vi "Subsequence Exchange Crossover(SXX).vi"(8 "Number of Jobs":i32, 9 "Number of Machines":i32, 10 "Schedule 2":u16[](array[numeric]), 11 "Schedule 1":u16[](array[numeric])) -> (2 "Child 2":T1, 3 "Child 1":T1)   [LabVIEW 2013, in "GA.lvclass"]
uses:
  GA.lvclass
  Controls/Subsequence.ctl
  Controls/Appropraite Subsequences for SXX.ctl
  Controls/Solution_GA.ctl
  <vilib>/Analysis/NI_AALBase.lvlib
  <vilib>/Analysis/1siggen.llb/Riffle Array (I32).vi
panel:
  out "Schedule 2":u16[](array[numeric])
  out "Schedule 1":u16[](array[numeric])
  out "Appropriate Subsequences":T2[](array[typedef])
  out "All Subarrays Out 2":T3[](array[typedef])
  out "All Subarrays Out 1":T3[](array[typedef])
  out "JO4M Sch2":u16[][](array[numeric])
  out "JO4M Sch1":u16[][](array[numeric])
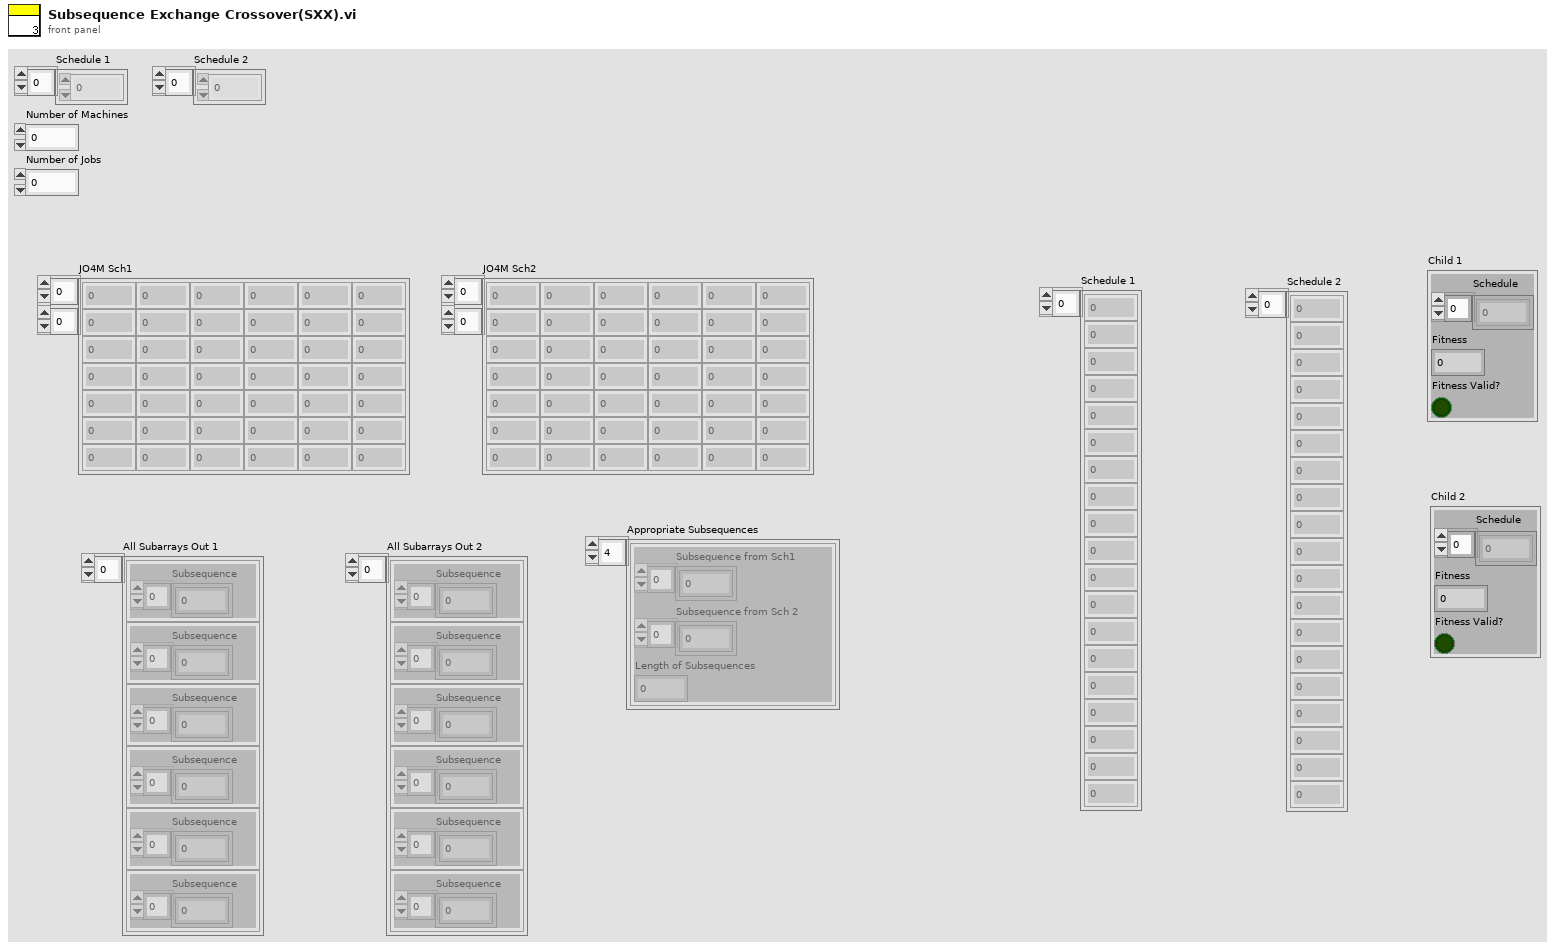
[diagram p1: front panel]
types:
  T1 = typedef "Solution_GA.ctl" = cluster{"Schedule":u16[], "Fitness":u16, "Fitness Valid?":bool}
  T2 = typedef "Appropraite Subsequences for SXX.ctl" = cluster{"Subsequence from Sch1":i32[], "Subsequence from Sch 2":i32[], "Length of Subsequences":i32}
  T3 = typedef "Subsequence.ctl" = cluster{"Subsequence":i32[]}
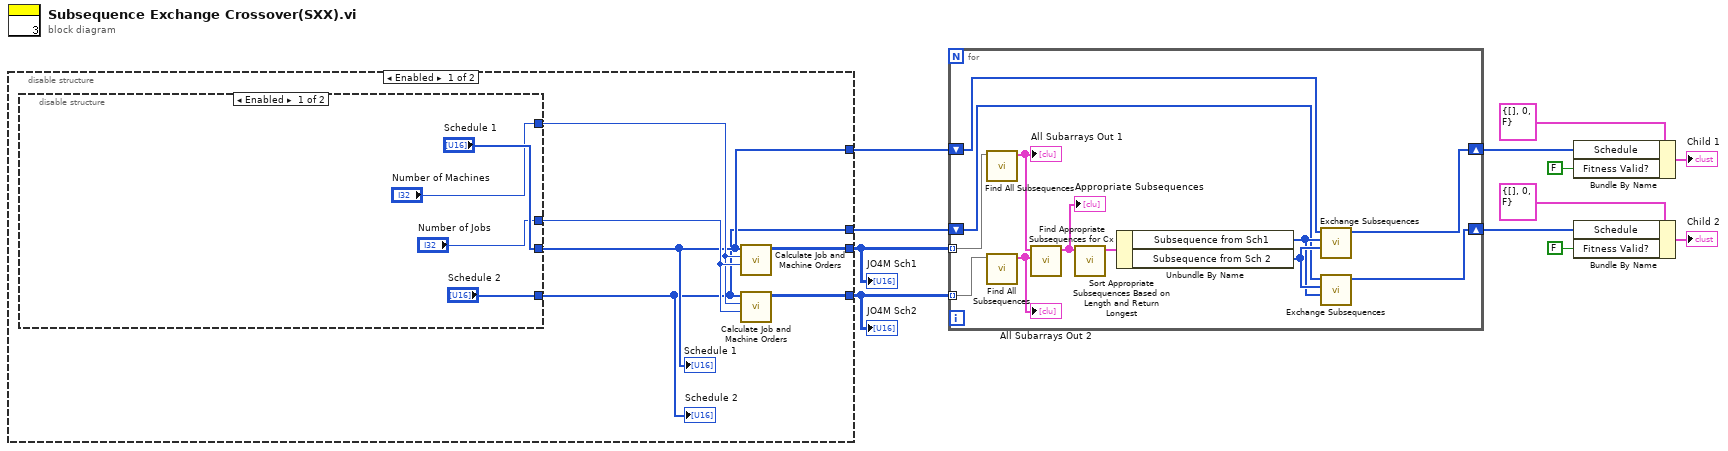
[diagram p0: block diagram]
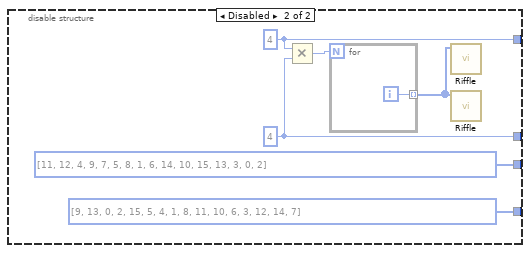
[diagram p2: hidden frame]
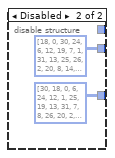
[diagram p3: hidden frame]
diagram:
  n1 = disable-structure shown="Enabled" {
    disable-tunnel: [w16 u16[][] [[18, 0, 30, 24, 6, 12], [19, 7, 1, 31, 13, 25], [26, 2, 20, 8, 14, 32], [33, 27, 15, 3, 21, 9], [34, 28, 10, 4, 16, 22], [29, 35, 11, 17, 5, 23]] ("JO4M Sch1")] -> w12
    disable-tunnel: [w15 u16[][] [[30, 18, 0, 6, 24, 12], [1, 25, 19, 13, 31, 7], [8, 26, 20, 2, 14, 32], [27, 9, 3, 21, 15, 33], [16, 28, 22, 34, 10, 4], [5, 17, 29, 11, 35, 23]] ("JO4M Sch2")] -> w11
    disable-tunnel: [w14 _] -> w10
    disable-tunnel: [w13 _] -> w9
    frame Enabled {
      n2 = disable-structure shown="Enabled" {
        disable-tunnel: ["Schedule 1" i32[] [11, 12, 4, 9, 7, 5, 8, 1, 6, 14, 10, 15, 13, 3, 0, 2] ("Schedule 1")] -> w14
        disable-tunnel: ["Schedule 2" i32[] [9, 13, 0, 2, 15, 5, 4, 1, 8, 11, 10, 6, 3, 12, 14, 7] ("Schedule 2")] -> w13
        disable-tunnel: ["Number of Jobs" w27] -> w18
        disable-tunnel: ["Number of Machines" w28] -> w17
        frame Enabled {
        }
        frame Disabled {
          w27 = 4 ("Number of Jobs")
          w28 = 4 ("Number of Machines")
          n3 = Multiply(x=w28, y=w27) -> (x*y=w26:i32)
          n4 = for {
            N: w26 -> [_]
            tunnel: [w29] -> w25 mode=indexing
            i -> [w29]
          }
          n5 = call-poly <vilib>:"Riffle.vi"("X"=w25) -> ()  [unwired: 8 in, 3 out]
          n6 = call-poly <vilib>:"Riffle.vi"("X"=w25) -> ()  [unwired: 8 in, 3 out]
        }
      }
      "Schedule 1" <- w14
      "Schedule 2" <- w13
      n7 = call "Calculate Job and Machine Orders.vi"("Number of Jobs"=w18, "Number of Machines"=w17, "Schedule"=w14) -> ("JO4M"=w16:u16[][])  [unwired: 7 in, 1 out]
      n8 = call "Calculate Job and Machine Orders.vi"("Number of Jobs"=w18, "Number of Machines"=w17, "Schedule"=w13) -> ("JO4M"=w15:u16[][])  [unwired: 7 in, 1 out]
    }
    frame Disabled {
    }
  }
  "JO4M Sch1" <- w12
  "JO4M Sch2" <- w11
  n9 = for {
    tunnel: w12 -> [w43] mode=indexing
    tunnel: w11 -> [w42] mode=indexing
    shift-right: [w38] -> w6
    shift-left: w10 -> [w36]
    shift-right: [w32] -> w3
    shift-left: w9 -> [w33]
    n10 = call "Find All Subsequences.vi"("JO4M"=w43) -> ("All Subarrays Out"=w41:T3[])  [unwired: 10 in]
    "All Subarrays Out 1" <- w41
    n11 = call "Find All Subsequences.vi"("JO4M"=w42) -> ("All Subarrays Out"=w40:T3[])  [unwired: 10 in]
    "All Subarrays Out 2" <- w40
    n12 = call "Find Appropriate Subsequences for Cx.vi"("All Subarrays Out 2"=w40, "All Subarrays Out 1"=w41) -> ("Appropriate Subsequences"=w39:T2[])  [unwired: 9 in]
    "Appropriate Subsequences" <- w39
    n13 = call "Sort Appropriate Subsequences Based on Length and Return Longest.vi"("Appropriate Subsequences"=w39) -> ("Logest Length Subsequence Match"=w37:T2)  [unwired: 10 in]
    n14 = Unbundle By Name(w37) -> ("Subsequence from Sch1"=w34:i32[], "Subsequence from Sch 2"=w35:i32[])
    n15 = call "Exchange Subsequences.vi"("Subsequence 2"=w35, "Subsequence 1"=w34, "Schedule In"=w36) -> ("Child Out"=w38:u16[])  [unwired: 8 in]
    n16 = call "Exchange Subsequences.vi"("Subsequence 2"=w34, "Subsequence 1"=w35, "Schedule In"=w33) -> ("Child Out"=w32:u16[])  [unwired: 8 in]
  }
  n17 = Bundle By Name(cluster=T1 {"Schedule"=[], "Fitness"=0, "Fitness Valid?"=FALSE} ("input cluster"), "Schedule"=w6, "Fitness Valid?"=FALSE) -> (→"Child 1":T1)
  n18 = Bundle By Name(cluster=T1 {"Schedule"=[], "Fitness"=0, "Fitness Valid?"=FALSE} ("input cluster"), "Schedule"=w3, "Fitness Valid?"=FALSE) -> (→"Child 2":T1)
